vi "Database Connection small.vi"(8 "error in (no error)":errorcluster) -> (0 "error out":errorcluster)   [LabVIEW 2013]
uses:
  Post_Dust_Event_small.ctl
  Private/Controls/File_location.ctl
  Public API/DisplayExperimentSetting.ctl
  Private/Controls/dust type.ctl
  Private/Controls/source_builders.ctl
  Private/Controls/Operator.ctl
  Private/Controls/dust_type_indicator.ctl
  <vilib>/Utility/miscctls.llb/LVPointTypeDef.ctl
  Public API/Dust_Event.ctl
  Public API/Signal.ctl
  Private/Controls/Role ID.ctl
  Private/Controls/Hardware ID.ctl
  Private/Controls/Estimate_source.ctl
  <vilib>/Utility/error.llb/DialogType.ctl
  Functional Global Variables/Action Items.ctl
  Private/UI Elements/throttle.vi
  Private/Sub-Polymorphic/post_dust_event_small.vi
panel:
  out "Experiment Settings Error":errorcluster
  out "Dust Processing error":errorcluster
  in  "Default Experiment Name":string="NDA" caption="Please Enter Tags:"
  in  "default Experiment Description":string="Database testing during NDA run in August." caption="Please Enter Experiment Description:"
  in  "Default Group ID":u16(ring)=3 items=["CCLDAS"=1, "LASP"=2, "CU"=3, "NLSI"=4, "LDEX"=5, "Heidelberg"=6]
  in  "Tab Control":enum32{"Status", "Processing", "Error Handling"}(tab)
  out "Dust Properties":T1
  in  "Update dust info":bool
  in  "Update Experiment Settings":bool
  out "output cluster 2":T2={"Current Experiment Name:"="NDA", "Current Experiment Description:"="Database testing during NDA run in August.", "Current Experiment Group ID:"="Database Testing", "Experiment Settings Last Updated At:"=timestamp(3427974586.5021 s since 1904-01-01)}
  out "Dust Type":T3 {"Batch" step=1; "Type" step=1; "Dust Source Builder:" items=["Keith Drake", "Nick Beaty", "Anthony Shu", "David James", "John Fontanese"]}
  out "# Events posted during current session:":i32=96
  out "# Events in dust event queue:":i32=388
  in  "Update Operator":bool
  out "Current Operator:":T5 {"Operator" items=["Giraffe", "Andrew Collette", "Keith Drake", "Anthony Shu", "Evan Thomas", "Nicholaus Beaty", "David James", "John Fontanese", ""]}
  out "Dust Event Processing:":T6={"Dust Event ID"=0, "Integer Timestamp"=13461087072182, "Velocity"=nan, "Mass"=nan, "Charge"=2.2111935e-15, "Radius"=0.0, "Needle Voltage (MV)"=0.0, "Experiment Settings"=0.0, "Estimate Quality"=0.0, "File Location"=0, "id_dust_info"=0.0} {"File Location" items=["Unknown"=-1, "Processing"=0, "Storage"=1]}
  in  "Write Signals":bool=TRUE
  out "Test":bool caption="Test Database in use:"
  out "Test 2":bool=TRUE caption="Production Database in use:"
  in  "Exit":bool=TRUE
  # "CCLDAS Database Connection for Small Accelerator \nV2.1.0"
  # "Experiment Status:"
  # "Dust Information"
  # "Queue Status:"
  # "Dust Event Small"
  # "ODBC Connection Status:"
  # "Error Status:"
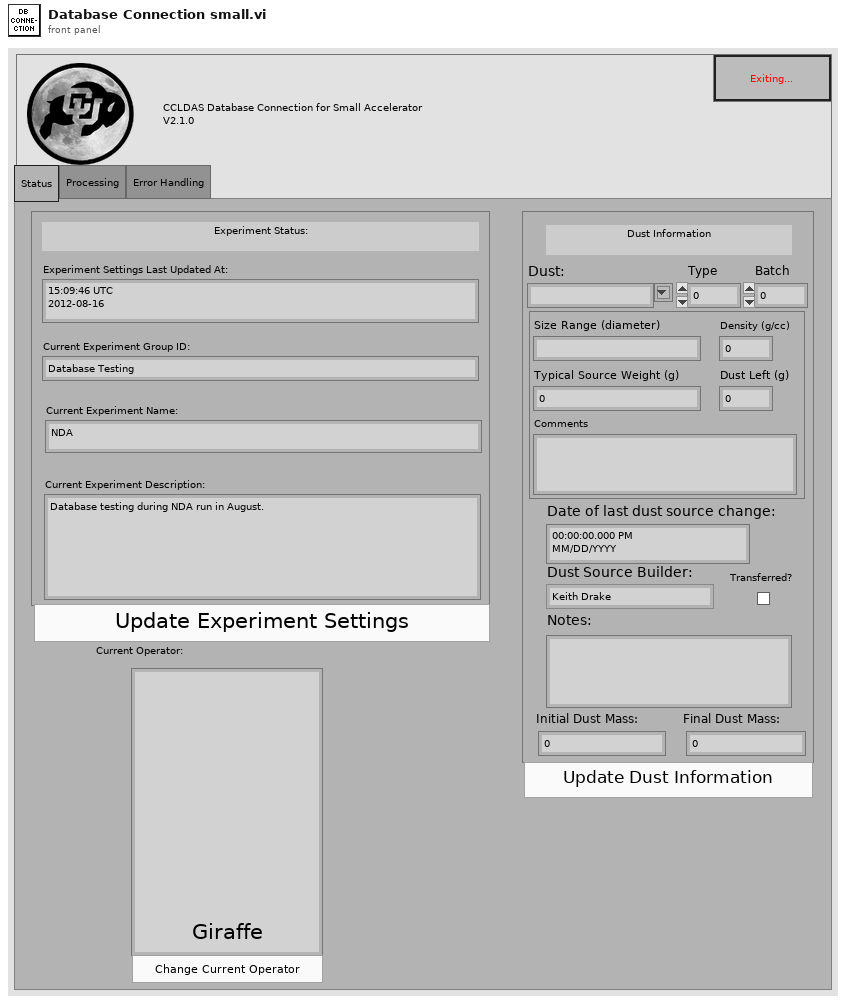
[diagram p1: front panel]
types:
  T1 = typedef "dust_type_indicator.ctl" = cluster{"Size Range (diameter)":string, "Density (g/cc)":dbl, "Typical Source Weight (g)":dbl, "Dust Left (g)":dbl, "Comments":string}
  T2 = typedef "DisplayExperimentSetting.ctl" = cluster{"Current Experiment Name:":string, "Current Experiment Description:":string, "Current Experiment Group ID:":string, "Experiment Settings Last Updated At:":timestamp}
  T3 = typedef "dust type.ctl" = cluster{"Dust info id":u16, "Integer Timestamp":i64, "Dust:":string, "Dust Source Builder:":T4, "Notes:":string, "Date of last dust source change:":timestamp, "Initial Dust Mass:":dbl, "Final Dust Mass:":dbl, "Type":u16, "Batch":u16, "dust type id":u16, "Transferred?":bool}
  T4 = typedef "source_builders.ctl" = u16
  T5 = typedef "Operator.ctl" = cluster{"Timestamp":i64, "Operator":u16}
  T6 = typedef "Post_Dust_Event_small.ctl" = cluster{"Dust Event ID":i64, "Integer Timestamp":i64, "Velocity":sgl, "Mass":sgl, "Charge":sgl, "Radius":sgl, "Needle Voltage (MV)":dbl, "Experiment Settings":dbl, "Estimate Quality":sgl, "File Location":T7, "id_dust_info":dbl}
  T7 = typedef "File_location.ctl" = i8
  T8 = typedef "LVPointTypeDef.ctl" = cluster{"Horizontal":i16, "Vertical":i16}
  T9 = typedef "Dust_Event.ctl" = cluster{"Time Stamp":timestamp, "Velocity":sgl, "Mass":sgl, "Charge":sgl, "Radius":sgl, "Array":T10[], "Dust Event ID":i64, "Passed_3rd_Detector":bool, "Estimate Source":T13, "Estimate Quality":sgl}
  T10 = typedef "Signal.ctl" = cluster{"Signal ID":i64, "Time Stamp":timestamp, "Dust Event ID":i64, "Role ID":T11, "Data":sgl[], "Signal Length":i32, "dt":sgl, "Offset":dbl, "Hardware ID":T12}
  T11 = typedef "Role ID.ctl" = enum16{"First_Detector", "Second_Detector", "Third_Detector", "LeCroy_CH1", "LeCroy_CH2", "LeCroy_CH3", "LeCroy_CH4", "PSU"}
  T12 = typedef "Hardware ID.ctl" = enum16{"Unknown", "CSA 1", "CSA 2", "CSA 3", "CSA 4", "CSA 5", "CSA 6"}
  T13 = typedef "Estimate_source.ctl" = i8
  T14 = typedef "Action Items.ctl" = enum16{"Initialize", "Get", "Set"}
  T15 = typedef "DialogType.ctl" = u16
  T16 = typedef "NI_Database_API.lvlib/Conn ObjectReference.ctl" = refnum<k1>
  T17 = typedef "Semaphore RefNum" = refnum<k1>
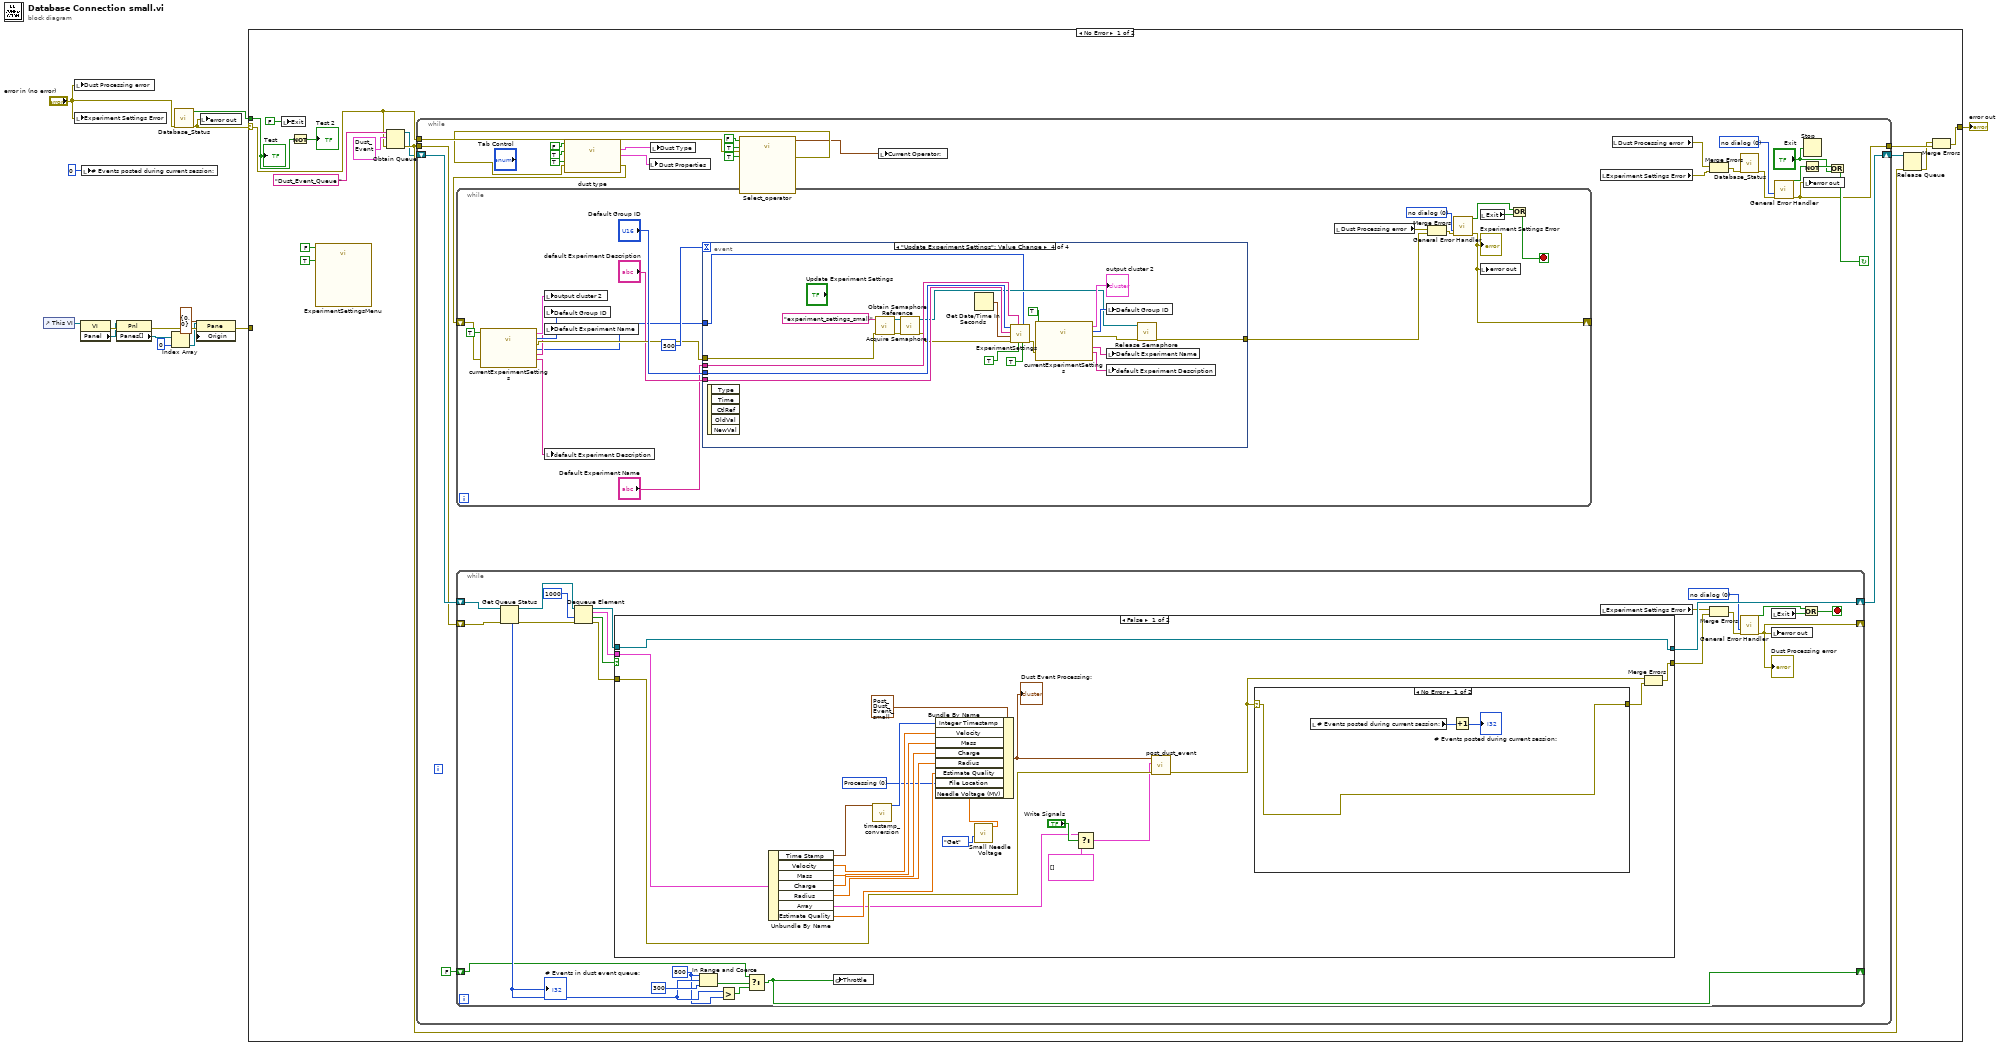
[diagram p0: block diagram]
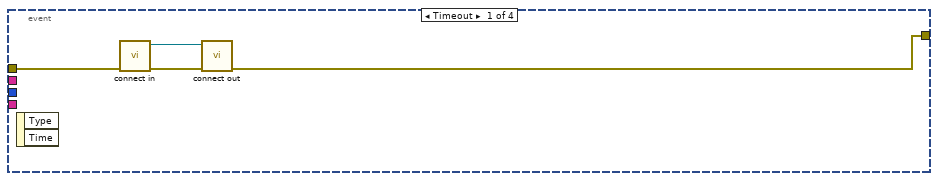
[diagram p2: hidden frame]
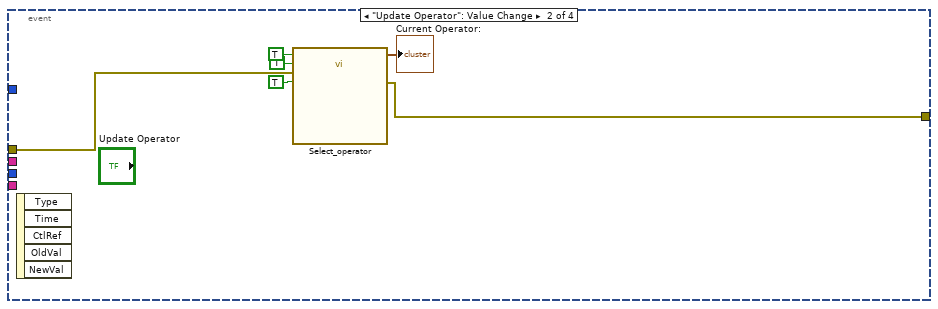
[diagram p3: hidden frame]
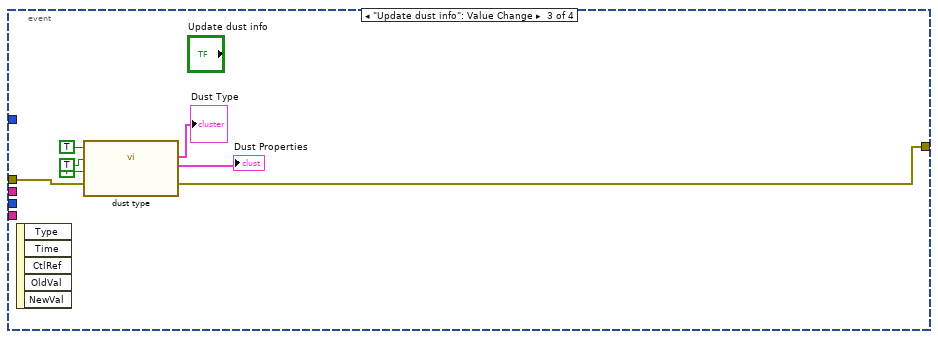
[diagram p4: hidden frame]
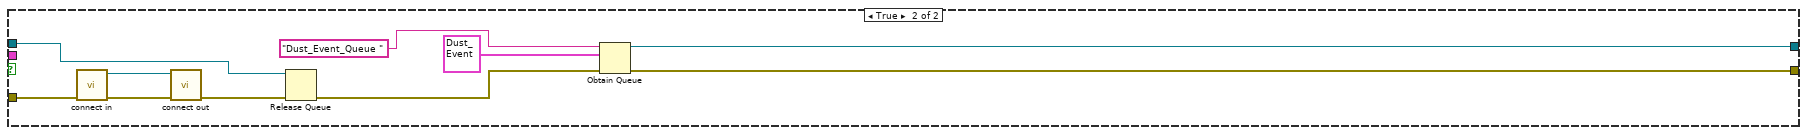
[diagram p6: hidden frame]
diagram:
  n1 = control-ref of="This VI"() -> (w9:refnum<vi>)
  n2 = local write "Dust Processing error"("error in (no error)") -> ()
  n3 = local write "Experiment Settings Error"("error in (no error)") -> ()
  n4 = property class="VI"(reference=w9) -> (error out=w8:errorcluster, "Panel"=w7:refnum<vi>)  [unwired: 1 in, 1 out]
  n5 = local write "# Events posted during current session:"(0) -> ()
  n6 = property class="Pnl"(reference=w7, error in=w8) -> (error out=w6:errorcluster, "Panes[]"=w5:refnum<vi>[])  [unwired: 1 out]
  n7 = Index Array(array=w5, index=0) -> (element=w3:refnum<vi>)
  n8 = call "Database_Status.vi"("error in (no error)"="error in (no error)") -> ("error out"=w12:errorcluster, "Test Database"=w14:bool)  [unwired: 9 in]
  n9 = property class="Pane"(reference=w3, error in=w6, "Origin"=T8 {"Horizontal"=0, "Vertical"=0}) -> (error out=w1:errorcluster)  [unwired: 1 out]
  n10 = local write "error out"(w12) -> ()
  n11 = case shown="No Error" w12 {
    selector: w12 -> [w18 w174]
    tunnel: [w17 w174] -> w13
    tunnel: w14 -> [w19 _]
    tunnel: w1 -> [_ _]
    frame No Error {
      n12 = local write "Exit"(FALSE ("Exit")) -> ()
      n13 = Not(x=w19) -> (.not. x?=→"Test 2":bool)
      n14 = call "ExperimentSettingsMenu.vi"("Enable"=FALSE, "sub vi?"=TRUE) -> ()  [unwired: 11 in, 7 out]
      n15 = Obtain Queue(name (unnamed)="Dust_Event_Queue ", element data type=T9 {"Time Stamp"=timestamp(0 s since 1904-01-01), "Velocity"=0.0, "Mass"=0.0, "Charge"=0.0, "Radius"=0.0, "Array"=[], "Dust Event ID"=0, "Passed_3rd_Detector"=FALSE, "Estimate Source"=0, "Estimate Quality"=0.0} ("Cluster"), error in (no error)=w18) -> (queue out=w22:refnum<queue>, error out=w24:errorcluster)  [unwired: 2 in, 1 out]
      n16 = while {
        tunnel: w24 -> [w52]
        tunnel: [w47] -> w28
        tunnel: w18 -> [w39]
        shift-right: [w53] -> w23
        shift-left: w22 -> [w54]
        stop <- w50 continue-if-true
        w44 = T15 0 items=["no dialog", "OK message", "continue or stop message", "OK message + warnings", "continue/stop + warnings"] ("type of dialog (OK msg:1)")
        n17 = while {
          shift-right: [w123] -> _
          shift-left: w52 -> [w136]
          shift-right: [w135] -> w53
          shift-left: w54 -> [w137]
          shift-right: [w113] -> _
          shift-left: FALSE -> [w115]
          stop <- w131 stop-if-true
          w117 = 800 ("y")
          w133 = T15 0 items=["no dialog", "OK message", "continue or stop message", "OK message + warnings", "continue/stop + warnings"] ("type of dialog (OK msg:1)")
          n18 = Get Queue Status(queue=w137, error in (no error)=w136) -> (queue out=w129:refnum<queue>, error out=w127:errorcluster, # elements in queue=w118:i32)  [unwired: 1 in, 5 out]
          "# Events in dust event queue:" <- w118
          n19 = Dequeue Element(queue=w129, timeout in ms (-1)=u32 1000 ("milliseconds to wait"), error in (no error)=w127) -> (queue out=w128:refnum<queue>, element=w130:T9, timed out?=w125:bool, error out=w126:errorcluster)
          n20 = case shown="False" w125 {
            tunnel: w128 -> [w151 w167]
            tunnel: w126 -> [w146 w173]
            tunnel: [w151 w165] -> w135
            tunnel: [w147 w164] -> w122
            tunnel: w130 -> [w150 _]
            frame False {
              w138 = T7 0 items=["Unknown"=-1, "Processing"=0, "Storage"=1] ("File Location")
              n21 = Unbundle By Name(w150) -> ("Time Stamp"=w158:timestamp, "Velocity"=w154:sgl, "Mass"=w155:sgl, "Charge"=w156:sgl, "Radius"=w157:sgl, "Array"=w142:T10[], "Estimate Quality"=w149:sgl)
              n22 = call "timestamp_conversion.vi"("Time Stamp"=w158) -> ("Integer Time"=w159:i64)  [unwired: 8 in, 1 out]
              n23 = call "Small Needle Voltage.vi"("Action"=Action_Items."Get") -> ("Output Pelletron Voltage"=w144:dbl)  [unwired: 10 in]
              n24 = Bundle By Name(cluster=T6 {"Dust Event ID"=0, "Integer Timestamp"=0, "Velocity"=0.0, "Mass"=0.0, "Charge"=0.0, "Radius"=0.0, "Needle Voltage (MV)"=0.0, "Experiment Settings"=0.0, "Estimate Quality"=0.0, "File Location"=0, "id_dust_info"=0.0} ("Cluster 2"), "Integer Timestamp"=w159, "Velocity"=w154, "Mass"=w155, "Charge"=w156, "Radius"=w157, "Estimate Quality"=w149, "File Location"=w138, "Needle Voltage (MV)"=w144) -> (w152:T6)
              "Dust Event Processing:" <- w152
              n25 = Select(t=w142, s="Write Signals", f=T10[] []) -> (s? t:f=w140:T10[])
              n26 = call-poly "post_dust_event.vi"("error in (no error)"=w146, "Signal Array"=w140, "Cluster"=w152) -> ("error out"=w141:errorcluster)  [unwired: 5 in, 3 out]
              n27 = case shown="No Error" w141 {
                selector: w141 -> [w160 w163]
                tunnel: [w160 w163] -> w148
                frame No Error {
                  n28 = local read "# Events posted during current session:"() -> (w162:i32)
                  n29 = Increment(x=w162) -> (x+1=→"# Events posted during current session:":i32)
                }
                frame Error {
                }
              }
              n30 = Merge Errors(w141, w148) -> (w147:errorcluster)
            }
            frame True {
              n31 = call "connect in.vi"("error in (no error)"=w173) -> ("error out"=w172:errorcluster, "Database Connection"=w171:T16)  [unwired: 6 in, 1 out]
              n32 = call "connect out.vi"("error in (no error)"=w172, "connection reference"=w171) -> ("error out"=w168:errorcluster)  [unwired: 9 in]
              n33 = Release Queue(queue=w167, error in (no error)=w168) -> (error out=w166:errorcluster)  [unwired: 1 in, 2 out]
              n34 = Obtain Queue(name (unnamed)="Dust_Event_Queue ", element data type=T9 {"Time Stamp"=timestamp(0 s since 1904-01-01), "Velocity"=0.0, "Mass"=0.0, "Charge"=0.0, "Radius"=0.0, "Array"=[], "Dust Event ID"=0, "Passed_3rd_Detector"=FALSE, "Estimate Source"=0, "Estimate Quality"=0.0} ("Cluster"), error in (no error)=w166) -> (queue out=w165:refnum<queue>, error out=w164:errorcluster)  [unwired: 2 in, 1 out]
            }
          }
          n35 = In Range and Coerce(upper limit=w117, x=w118, lower limit=300) -> (In Range?=w116:bool)  [unwired: 1 out]
          n36 = Greater?(x=w118, y=w117) -> (0:w114:bool)
          n37 = Select(t=w115, s=w116, f=w114) -> (s? t:f=w113:bool)
          n38 = global write "throttle.vi" "Throttle"(w113) -> ()
          n39 = local read "Experiment Settings Error"() -> (w120:errorcluster)
          n40 = Merge Errors(w120, w122) -> (w121:errorcluster)
          n41 = call <vilib>:"General Error Handler.vi"("type of dialog (OK msg:1)"=w133, "error in (no error)"=w121) -> ("error?"=w134:bool, "error out"=w123:errorcluster)  [unwired: 9 in, 3 out]
          "Dust Processing error" <- w123
          n42 = local read "Exit"() -> (w132:bool)
          n43 = local write "error out"(w123) -> ()
          n44 = Or(x=w134, y=w132) -> (x .or. y?=w131:bool)
        }
        n45 = call "Select_operator.vi"("Enable"=FALSE, "sub vi?"=TRUE, "error in (no error)"=w39, "small?"=TRUE) -> ("Operator Cluster 2"=w36:T5, "error out"=w38:errorcluster)  [unwired: 13 in, 1 out]
        n46 = call "dust type.vi"("Enable"=FALSE, "Small?"=TRUE, "Sub vi?"=TRUE, "error in (no error)"=w38) -> ("output cluster 2"=w41:T3, "Dust Properties 2"=w34:T1, "error out"=w42:errorcluster)  [unwired: 11 in, 2 out]
        n47 = while {
          shift-right: [w64] -> _
          shift-left: w42 -> [w66]
          stop <- w70 stop-if-true
          w72 = T15 0 items=["no dialog", "OK message", "continue or stop message", "OK message + warnings", "continue/stop + warnings"] ("type of dialog (OK msg:1)")
          n48 = call "currentExperimentSettings.vi"("small?"=TRUE, "error in (no error)"=w66) -> ("Last Name"=w61:string, "Last Description"=w60:string, "Experiment settings ID"=w56:i64, "output cluster"=w67:T2, "Last Group ID"=w68:i32, "error out"=w65:errorcluster)  [unwired: 12 in]
          n49 = local write "output cluster 2"(w67) -> ()
          n50 = local write "Default Group ID"(w68) -> ()
          n51 = local write "Default Experiment Name"(w61) -> ()
          n52 = local write "default Experiment Description"(w60) -> ()
          n53 = event shown="[3] \"Update Experiment Settings\": Value Change" {
            selector: _ -> [_ _ _ _]
            dyn-events: _ -> [_ _ _ _]
            timeout: 500 -> [_ _ _ _]
            tunnel: w65 -> [w76 w84 w89 w98]
            tunnel: [w75 w81 w90 w97] -> w59
            tunnel: "Default Group ID" -> [_ _ _ w110]
            tunnel: "default Experiment Description" -> [_ _ _ w109]
            tunnel: "Default Experiment Name" -> [_ _ _ w108]
            tunnel: w56 -> [_ _ _ w95]
            event Timeout {
              n54 = event-data() -> ()  [unwired: 1 in, 2 out]
              n55 = call "connect in.vi"("error in (no error)"=w76) -> ("error out"=w78:errorcluster, "Database Connection"=w77:T16)  [unwired: 6 in, 1 out]
              n56 = call "connect out.vi"("error in (no error)"=w78, "connection reference"=w77) -> ("error out"=w75:errorcluster)  [unwired: 9 in]
            }
            event "Update Operator": Value Change {
              n57 = event-data() -> ()  [unwired: 1 in, 5 out]
              n58 = call "Select_operator.vi"("Enable"=TRUE, "sub vi?"=TRUE, "error in (no error)"=w84, "small?"=TRUE) -> ("Operator Cluster 2"=→"Current Operator:":T5, "error out"=w81:errorcluster)  [unwired: 13 in, 1 out]
            }
            event "Update dust info": Value Change {
              n59 = event-data() -> ()  [unwired: 1 in, 5 out]
              n60 = call "dust type.vi"("Enable"=TRUE, "Small?"=TRUE, "Sub vi?"=TRUE, "error in (no error)"=w89) -> ("output cluster 2"=→"Dust Type":T3, "Dust Properties 2"=→"Dust Properties":T1, "error out"=w90:errorcluster)  [unwired: 11 in, 2 out]
            }
            event "Update Experiment Settings": Value Change {
              n61 = event-data() -> ()  [unwired: 1 in, 5 out]
              n62 = call <vilib>:"Obtain Semaphore Reference.vi"("error in (no error)"=w98, "name (unnamed)"="experiment_settings_small") -> ("error out"=w102:errorcluster, "semaphore"=w103:T17)  [unwired: 3 in, 1 out]
              n63 = call <vilib>:"Acquire Semaphore.vi"("error in (no error)"=w102, "semaphore"=w103) -> ("error out"=w94:errorcluster, "semaphore out"=w99:T17)  [unwired: 3 in, 1 out]
              n64 = Get Date/Time In Seconds() -> (seconds since 1Jan1904=w105:timestamp)
              n65 = call "ExperimentSettings.vi"("small?"=TRUE, "Experiment Settings id"=w95, "Enable"=TRUE, "Default Experiment Name"=w108, "error in (no error)"=w94, "current time"=w105, "default Experiment Description"=w109, "Default Group ID"=w110) -> ("error out"=w96:errorcluster)  [unwired: 2 in, 1 out]
              n66 = call "currentExperimentSettings.vi"("small?"=TRUE, "error in (no error)"=w96) -> ("Last Name"=w106:string, "Last Description"=w107:string, "output cluster"=→"output cluster 2":T2, "Last Group ID"=w111:i32, "error out"=w100:errorcluster)  [unwired: 12 in, 1 out]
              n67 = local write "Default Group ID"(w111) -> ()
              n68 = local write "Default Experiment Name"(w106) -> ()
              n69 = local write "default Experiment Description"(w107) -> ()
              n70 = call <vilib>:"Release Semaphore.vi"("error in (no error)"=w100, "semaphore"=w99) -> ("error out"=w97:errorcluster)  [unwired: 4 in, 1 out]
            }
          }
          n71 = local read "Dust Processing error"() -> (w57:errorcluster)
          n72 = Merge Errors(w57, w59) -> (w58:errorcluster)
          n73 = call <vilib>:"General Error Handler.vi"("type of dialog (OK msg:1)"=w72, "error in (no error)"=w58) -> ("error?"=w69:bool, "error out"=w64:errorcluster)  [unwired: 9 in, 3 out]
          "Experiment Settings Error" <- w64
          n74 = local read "Exit"() -> (w71:bool)
          n75 = local write "error out"(w64) -> ()
          n76 = Or(x=w69, y=w71) -> (x .or. y?=w70:bool)
        }
        n77 = local write "Dust Properties"(w34) -> ()
        n78 = local write "Dust Type"(w41) -> ()
        n79 = local write "Current Operator:"(w36) -> ()
        n80 = local read "Experiment Settings Error"() -> (w33:errorcluster)
        n81 = local read "Dust Processing error"() -> (w46:errorcluster)
        n82 = Merge Errors(w46, w33) -> (w45:errorcluster)
        n83 = call "Database_Status.vi"("error in (no error)"=w45) -> ("error out"=w51:errorcluster)  [unwired: 9 in, 1 out]
        n84 = call <vilib>:"General Error Handler.vi"("type of dialog (OK msg:1)"=w44, "error in (no error)"=w51) -> ("error?"=w43:bool, "error out"=w47:errorcluster)  [unwired: 9 in, 3 out]
        n85 = Not(x=w43) -> (.not. x?=w49:bool)
        n86 = Stop(stop? (T)="Exit") -> ()
        n87 = local write "error out"(w47) -> ()
        n88 = Or(x=w49, y="Exit") -> (x .or. y?=w50:bool)
      }
      n89 = Release Queue(queue=w23, error in (no error)=w24) -> (error out=w27:errorcluster)  [unwired: 1 in, 2 out]
      n90 = Merge Errors(w27, w28) -> (w17:errorcluster)
      "Test" <- w19
    }
    frame Error {
    }
  }
  "error out" <- w13
